vi "读取填充颜色.vi"(8 "error in (no error)":errorcluster caption="错误输入（无错误）", 11 "图形输入":refnum<class "图形.lvclass">) -> (0 "error out":errorcluster caption="错误输出", 2 "填充颜色":u32(colorbox), 3 "图形输出":refnum<class "图形.lvclass">)   [LabVIEW 2011, in "图形.lvclass"]
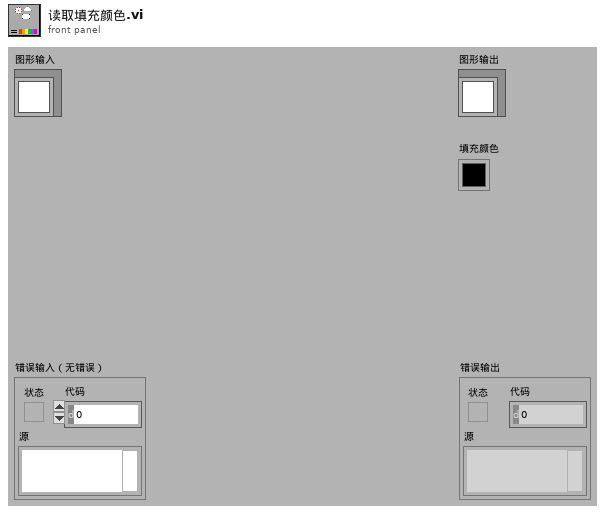
[diagram p1: front panel]
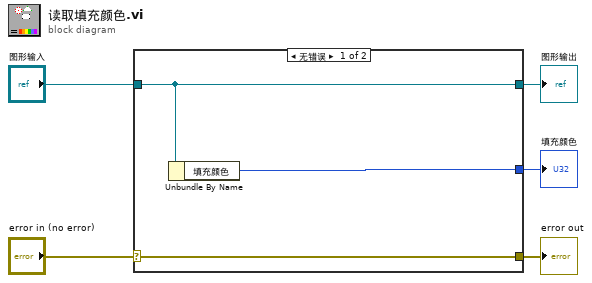
[diagram p0: block diagram]
diagram:
  n1 = case shown="无错误" "error in (no error)" {
    selector: "error in (no error)" -> [w8 w9]
    tunnel: [w8 w9] -> w4
    tunnel: [w7 w10] -> w2
    tunnel: "图形输入" -> [w7 w10]
    tunnel: [w6 _] -> w1
    frame No Error {
      n2 = Unbundle By Name(w7) -> ("填充颜色"=w6:u32)
    }
    frame Error {
    }
  }
  "error out" <- w4
  "图形输出" <- w2
  "填充颜色" <- w1
